vi "graphic_tester.vi"(11 "manager_daemon":refnum<class "manager_daemon.lvclass">=refnum) -> ()   [LabVIEW 2024]
uses:
  volume.type.colors--cluster.ctl
  comic_manager/manager_daemon/manager_daemon.lvclass
  selection_dropdown/Typedefs/Selection Dropdown.ctl
  selection_dropdown/selection_dropdown.lvclass/selection_dropdown.ctl
  <vilib>/Utility/miscctls.llb/LVPoint32TypeDef.ctl
  volume.object--cluster.ctl
  definitions/volume.type--enum.ctl
  comic_manager/TypeDefs/issue.display--cluster.ctl
  picture.data--cluster.ctl
  selection_dropdown/selection_dropdown.lvclass
  comic_manager/manager_daemon/manager_daemon.lvclass/manager_daemon.ctl
  comic_manager/TypeDefs/graphic.filter--cluster.ctl
  <vilib>/addons/_JKI Toolkits/State Machine/_JKI_lib_State_Machine.llb/Select State(s)_err__jki_lib_state_machine.vi
  <vilib>/addons/_JKI Toolkits/State Machine/_JKI_lib_State_Machine.llb/Periodic Trigger__ogtk__JKI-SM__jki_lib_state_machine.vi
panel:
  in  "concept filter":T1
  in  "storyArc filter":T1
  in  "character filter":T1
  in  "team filter":T1
  in  "Show Issues":bool=TRUE
  in  "Apply Filters":enum32{"AND", "OR"}(radio)
  in  "clear title":bool
  in  "title":string[](array[string])=["x-men", "x-factor", "x-force", "new mutants"]
  in  "Step Size":enum32{"Monthly", "Yearly"}(radio)
  in  "Show Legend":bool=TRUE
  in  "inc year":bool
  in  "dec year":bool
  in  "dec end year":bool
  in  "dec start year":bool
  in  "inc start year":bool
  in  "inc end year":bool
  in  "Legend":T2={"ongoing"=34559, "Limited Series"=35193, "Annuals"=16754450, "One Shots"=7566195, "Reprints"=16722176, "Star"=49407, "Epic"=8733439}
  in  "Plot End":timestamp=timestamp(3821234400 s since 1904-01-01) format="%<%x>T"
  in  "Plot Start":timestamp=timestamp(3537151200 s since 1904-01-01) format="%<%x>T"
  in  "Show All":bool=TRUE
  in  "Volume Type":T3={"Ongoing"=TRUE, "Limited Series"=TRUE, "Annuals"=TRUE, "One Shots"=TRUE, "Reference/Reprints"=TRUE, "Star Comics"=TRUE, "Epic Comics"=TRUE}
  out "volume":string
  out "found":i32=116
  in  "Exit":bool
  out "2D Picture":picture
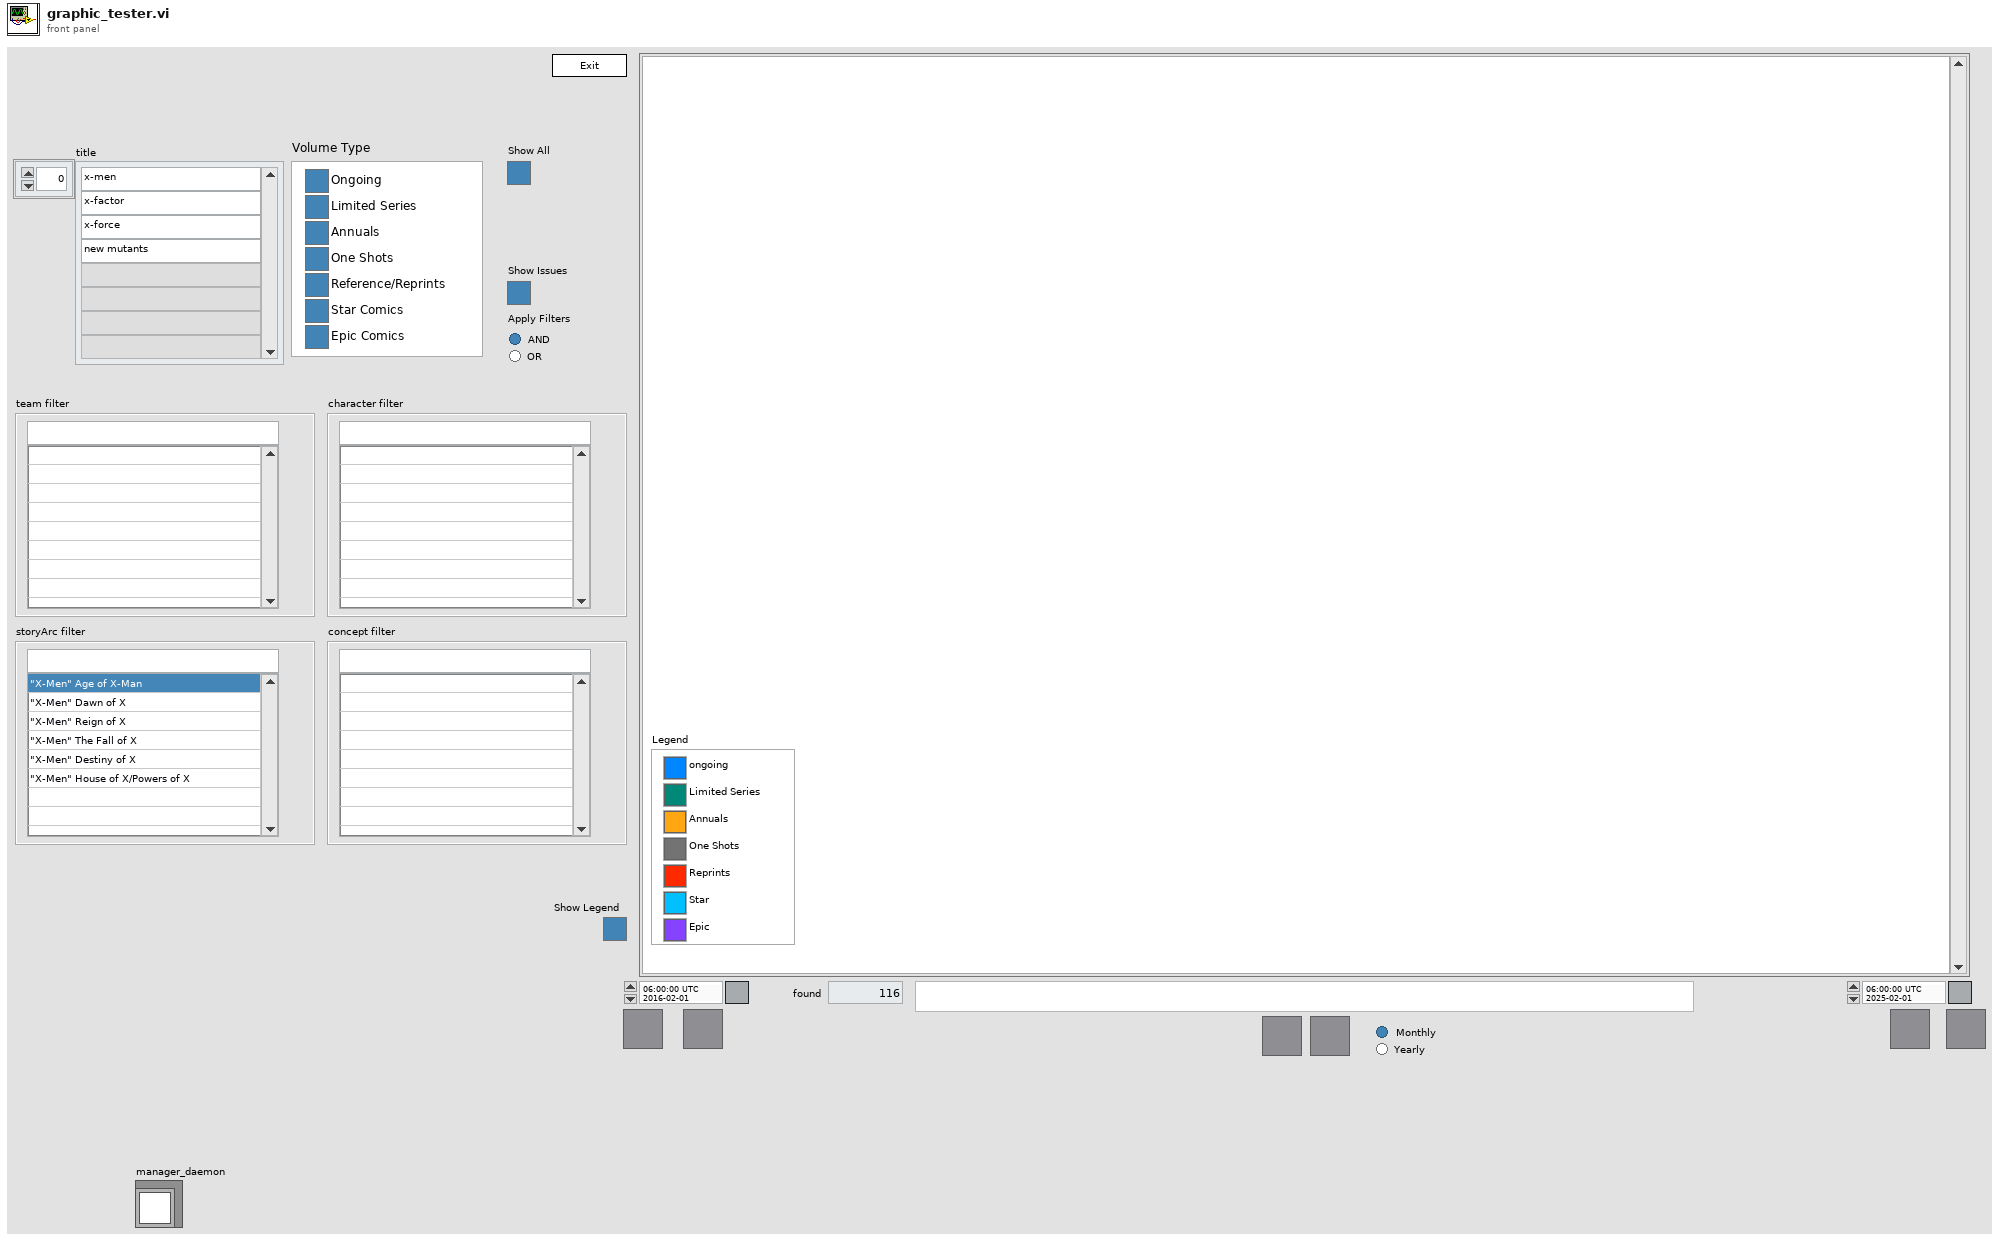
[diagram p1: front panel]
types:
  T1 = typedef "selection_dropdown.lvclass/Selection Dropdown.ctl" = cluster{"delete":bool, "available":i32, "list":i32, "cancel":bool, "selection":string, "delete all":bool}
  T2 = typedef "volume.type.colors--cluster.ctl" = cluster{"ongoing":u32, "Limited Series":u32, "Annuals":u32, "One Shots":u32, "Reprints":u32, "Star":u32, "Epic":u32}
  T3 = cluster{"Ongoing":bool, "Limited Series":bool, "Annuals":bool, "One Shots":bool, "Reference/Reprints":bool, "Star Comics":bool, "Epic Comics":bool}
  T4 = enum32{"Invalid", "Standard", "Closed", "Hidden", "Minimized", "Maximized"}
  T5 = enum32{"invalid app kind", "Development System", "Run Time System", "Student Edition", "Embedded LabVIEW", "Evaluation", "Custom"}
  T6 = typedef "graphic.filter--cluster.ctl" = cluster{"Volume Type":cluster{"Ongoing":bool, "Limited Series":bool, "Annuals":bool, "One Shots":bool, "Reference/Reprints":bool, "Star Comics":bool, "Epic Comics":bool}, "team":string[], "characters":string[], "storyArcs":string[], "Plot End":timestamp, "Plot Start":timestamp, "title":string[], "colors":T2, "concept":string[], "show all":bool, "Search by Title":enum32{"AND", "OR"}}
  T7 = cluster{"left":i16, "top":i16, "right":i16, "bottom":i16}
  T8 = typedef "volume.object--cluster.ctl" = cluster{"start date":timestamp, "end date":timestamp, "sortable_name":string, "color":u32, "volume type":T9, "issues":T10[]}
  T9 = typedef "volume.type--enum.ctl" = enum16{"Ongoing", "Limited Series", "Annual", "One Shot", "Reprint/Document", "Star Comics", "Epic Comics"}
  T10 = typedef "issue.display--cluster.ctl" = cluster{"cover_date":timestamp, "id":i32, "number":string, "fill":bool}
  T11 = typedef "picture.data--cluster.ctl" = cluster{"names":string[], "colors":u32[], "cells":cluster{"left":i16, "top":i16, "right":i16, "bottom":i16}[], "end date":timestamp, "start date":timestamp}
  T12 = typedef "LVPoint32TypeDef.ctl" = cluster{"Horizontal":i32, "Vertical":i32}
  T13 = cluster{"Core":cluster{"Current VI Reference":refnum<vi>, "Close Panel on Exit?":bool}, "volume objects":cluster{"Array":T8[]}[], "picture data":T11, "picture":picture, "rows":cluster{"left":i16, "top":i16, "right":i16, "bottom":i16}[], "cursor":T12, "manager_daemon":refnum<class "manager_daemon.lvclass">, "filters":cluster{"team filter":refnum<class "selection_dropdown.lvclass">, "story filter":refnum<class "selection_dropdown.lvclass">, "char filter":refnum<class "selection_dropdown.lvclass">, "concept filter":refnum<class "selection_dropdown.lvclass">}}
  T14 = typedef "LVPositionTypeDef.ctl" = cluster{"Left":i32, "Top":i32}
  T15 = cluster{"team filter":refnum<class "selection_dropdown.lvclass">, "story filter":refnum<class "selection_dropdown.lvclass">, "char filter":refnum<class "selection_dropdown.lvclass">, "concept filter":refnum<class "selection_dropdown.lvclass">}
  T16 = cluster{"left":i16, "top":i16, "right":i16, "bottom":i16}[]
  T17 = cluster{"Current VI Reference":refnum<vi>, "Close Panel on Exit?":bool}
  T18 = cluster{"team filter event":refnum<user-event>, "story filter event":refnum<user-event>, "char filter event":refnum<user-event>, "concept filter event":refnum<user-event>}
  T19 = typedef "LVBoundsTypeDef.ctl" = cluster{"Width":u32, "Height":u32}
  T20 = typedef "LVPointTypeDef.ctl" = cluster{"Horizontal":i16, "Vertical":i16}
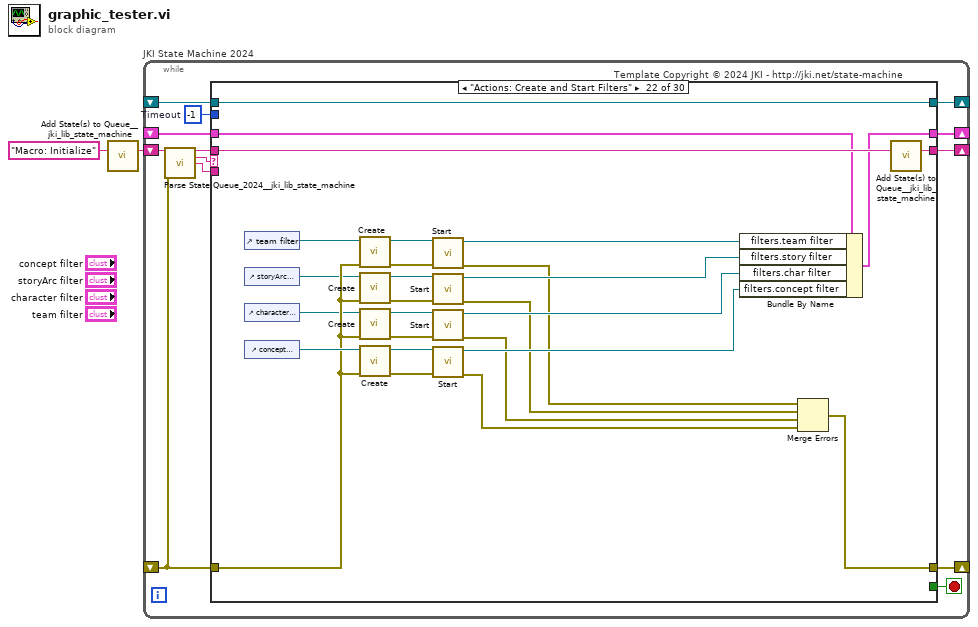
[diagram p0: block diagram]
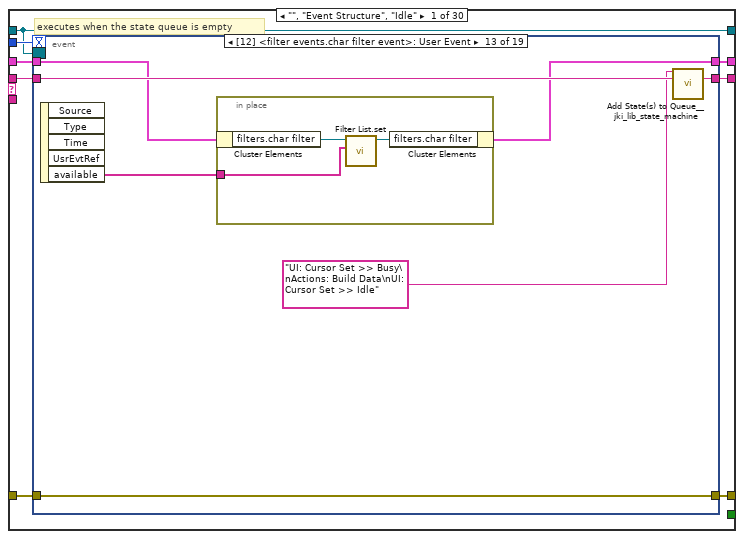
[diagram p2: hidden frame]
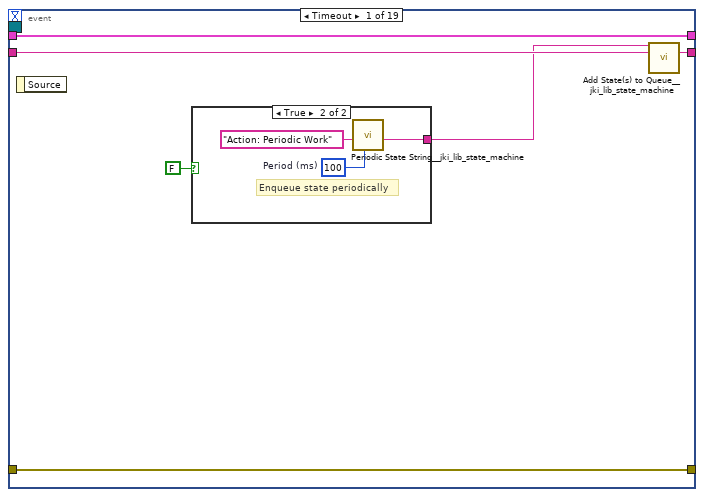
[diagram p3: hidden frame]
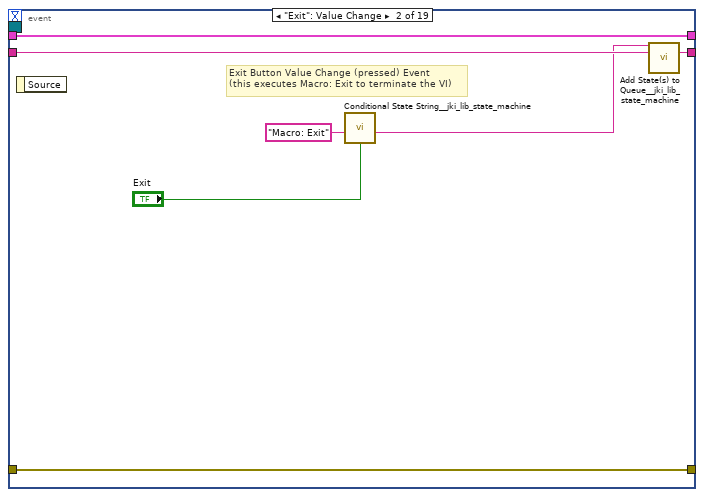
[diagram p5: hidden frame]
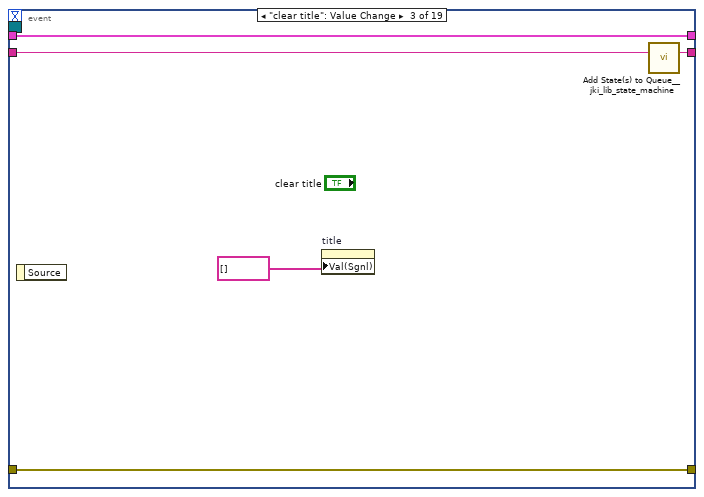
[diagram p6: hidden frame]
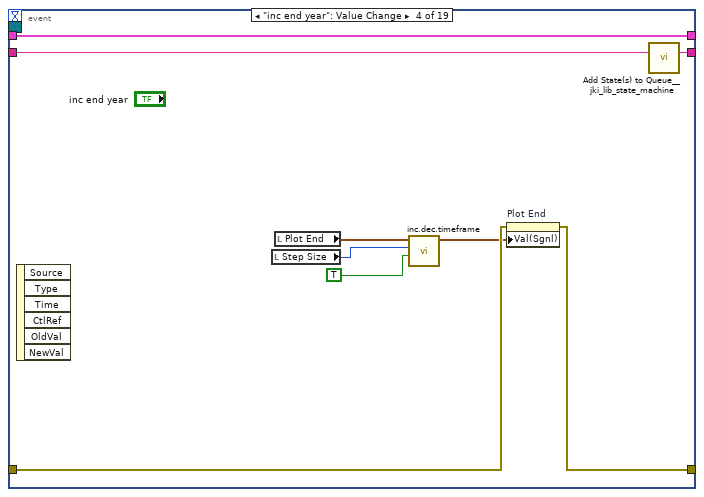
[diagram p7: hidden frame]
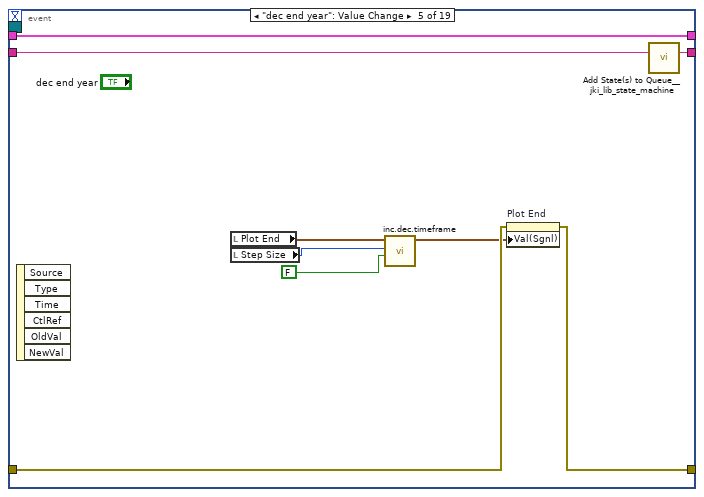
[diagram p8: hidden frame]
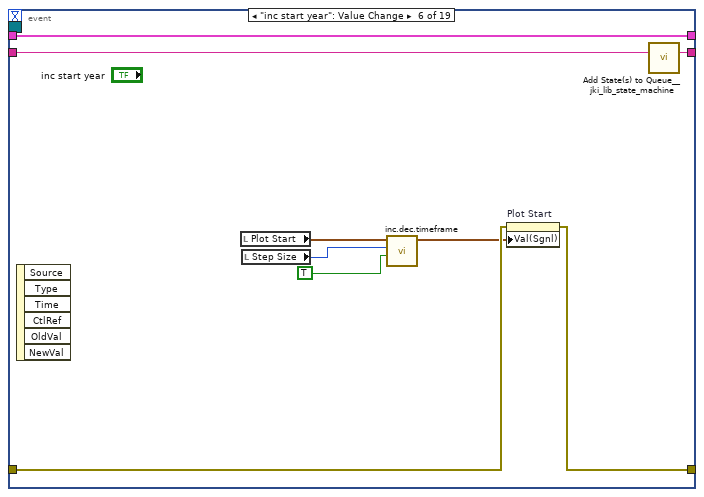
[diagram p9: hidden frame]
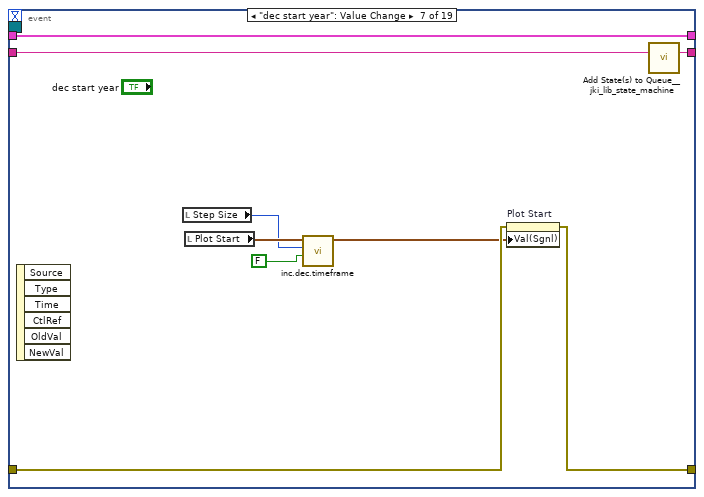
[diagram p10: hidden frame]
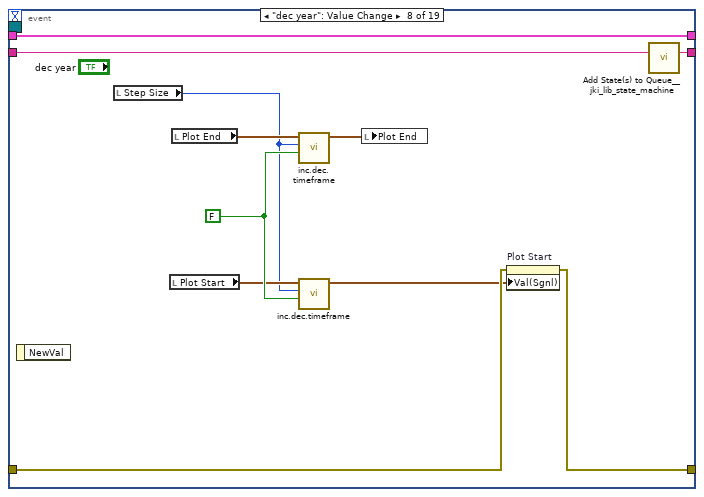
[diagram p11: hidden frame]
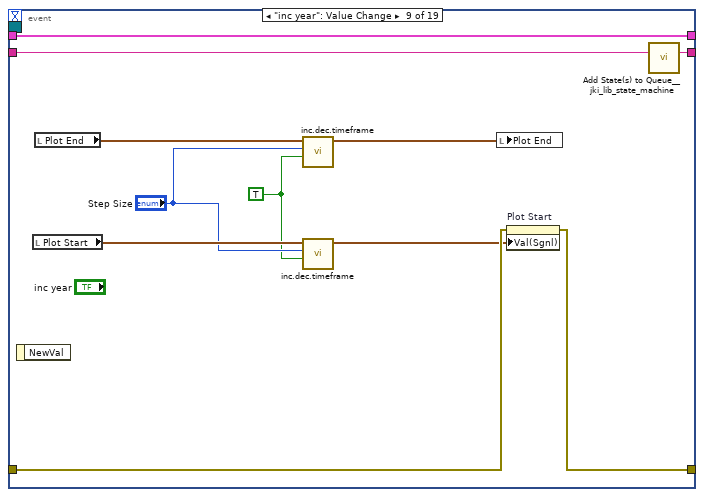
[diagram p12: hidden frame]
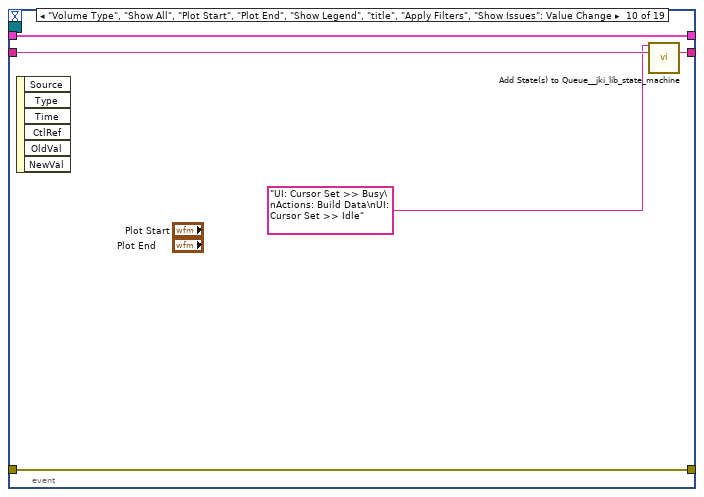
[diagram p13: hidden frame]
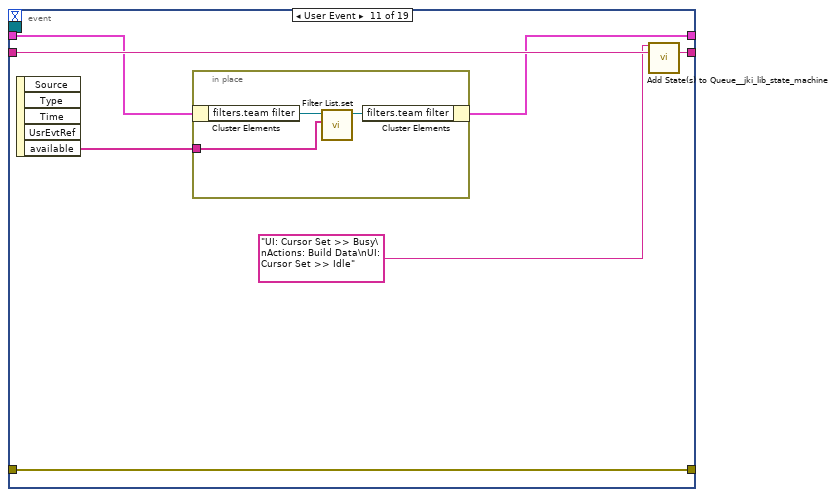
[diagram p14: hidden frame]
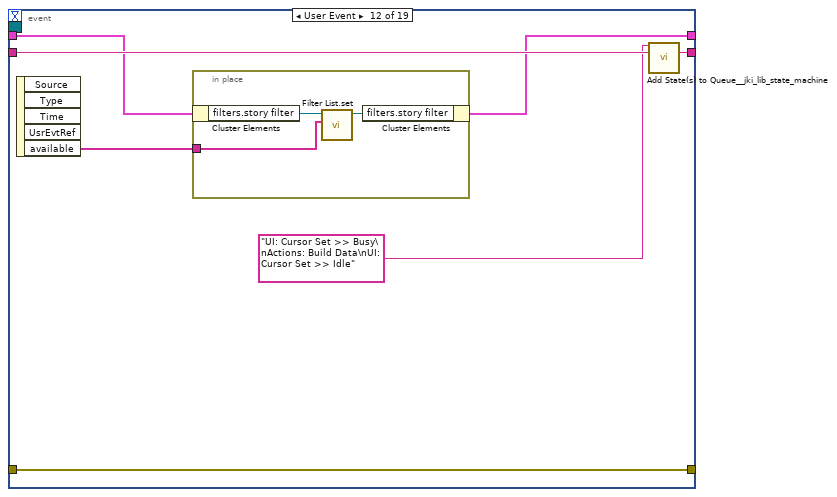
[diagram p15: hidden frame]
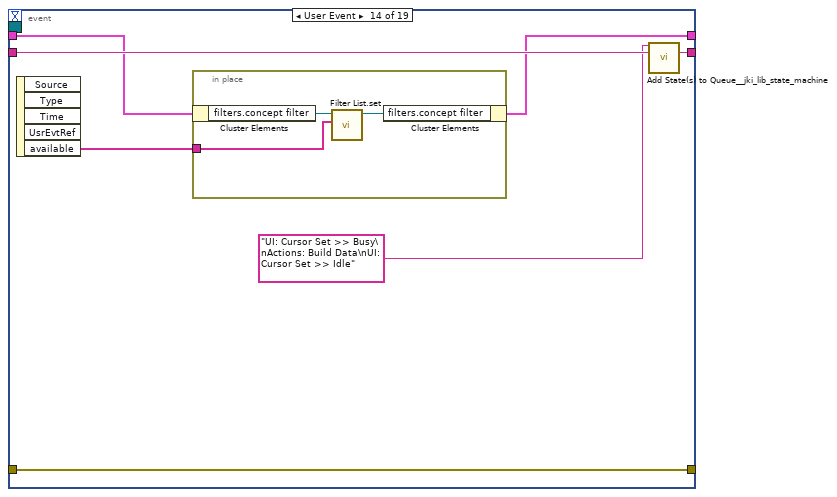
[diagram p16: hidden frame]
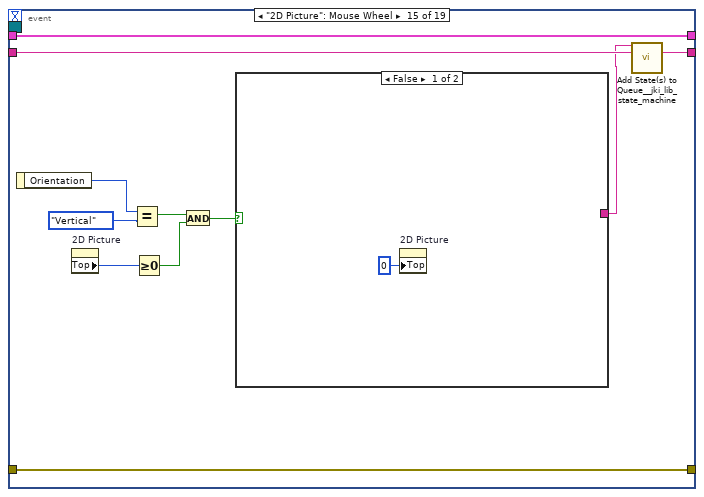
[diagram p17: hidden frame]
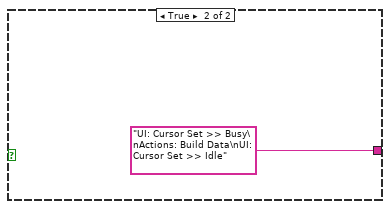
[diagram p18: hidden frame]
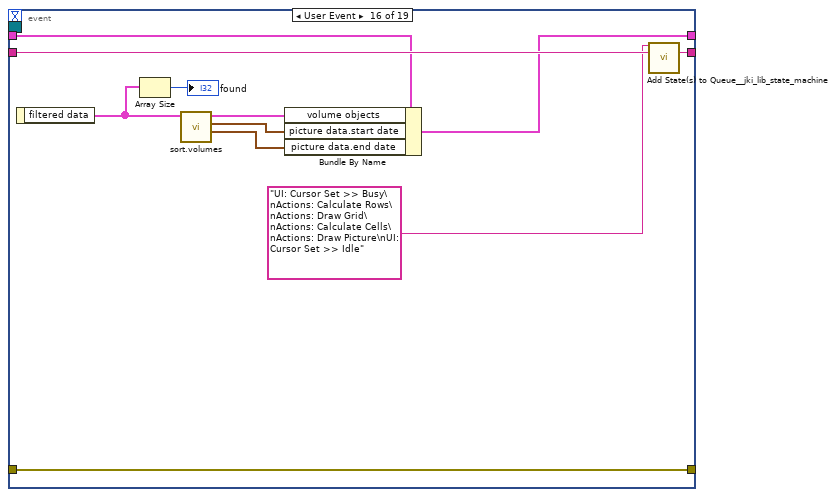
[diagram p19: hidden frame]
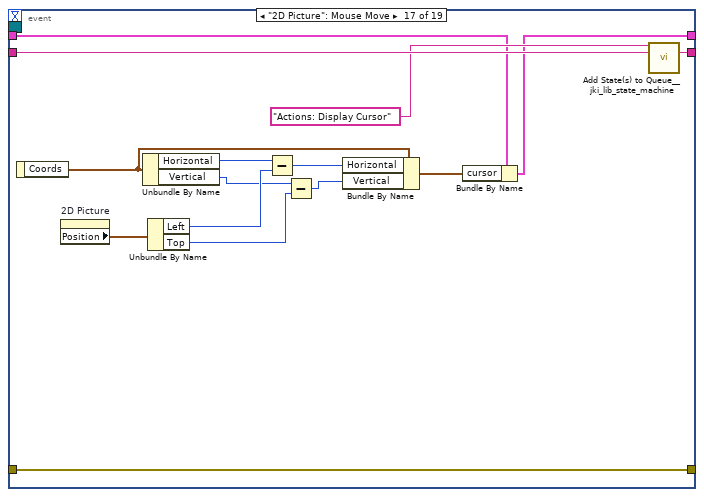
[diagram p20: hidden frame]
diagram:
  n1 = call <vilib>:"Add State(s) to Queue__jki_lib_state_machine.vi"("State(s) in (\"\")"="Macro: Initialize") -> ("States Out"=w2:string)  [unwired: 14 in]
  n2 = while "JKI State Machine 2024" {
    shift-right: [w8] -> _
    shift-left: _ -> [w7]
    shift-right: [w11] -> _
    shift-left: _ -> [w5]
    shift-right: [w10] -> _
    shift-left: w2 -> [w12]
    shift-right: [w4] -> _
    shift-left: _ -> [w3]
    stop <- w9 stop-if-true
    w6 = -1  # Timeout
    # "Template Copyright © 2024 JKI - http://jki.net/state-machine"
    n3 = call <vilib>:"Parse State Queue_2024__jki_lib_state_machine.vi"("State Queue"=w12, "Error In (no error)"=w5) -> ("Remaining States"=w14:string, "Current State"=w15:string, "Arguments"=w13:string)  [unwired: 11 in]
    n4 = case shown="\"Actions: Create and Start Filters\"" w15 {
      selector: w15 -> [_ _ w213 _ _ _ _ _ _ _ _ _ _ _ _ _ _ _ _ _ _ _ _ _ _ _ _ _ _ _]
      tunnel: w14 -> [w23 w211 w217 w237 w248 w258 w263 w281 w297 w302 w323 w329 w334 w339 w344 w351 w363 w433 w439 w449 w454 w481 w488 w497 w509 w521 w540 w565 w579 w603]
      tunnel: w13 -> [_ _ _ _ w243 _ _ _ _ _ _ _ _ _ _ w346 w357 _ _ _ _ _ _ _ _ _ _ _ _ _]
      tunnel: w7 -> [w21 w208 w215 w230 w245 w256 w260 _ w294 w299 w315 w327 w331 w337 w342 w349 w359 w430 w436 w447 w451 w465 w485 w495 w507 w518 w538 w556 w573 w594]
      tunnel: [w20 w209 w219 w234 errorcluster {"status"=FALSE, "code"=0, "source"=""} ("error out") w255 w261 w278 w287 w300 w316 w324 w332 w336 w341 w347 w360 w431 w437 w444 w452 w474 w482 w492 w504 w519 w535 w555 w577 w602] -> w11
      tunnel: w5 -> [w17 w209 w218 w234 w244 w255 w261 w278 w288 w300 w318 w325 w332 w336 w341 w348 w361 w431 w437 w444 w452 w466 w483 w494 w506 w519 w536 w554 w577 w602]
      tunnel: [w22 w210 w216 w236 w247 w257 w262 w280 w296 w301 w322 w328 w333 w338 w343 w350 w362 w432 w438 w448 w453 w480 w487 w496 w508 w520 w539 w564 w578 w603] -> w10
      tunnel: [_ _ _ _ _ TRUE _ _ _ _ _ _ _ _ _ _ _ _ _ _ _ _ _ _ _ _ _ _ _ _] -> w9
      tunnel: [w19 w208 w215 w235 w245 w256 w260 w279 w294 w299 w315 w327 w331 w337 w342 w349 w359 w430 w436 w447 w451 w475 w484 w495 w502 w518 w538 w556 w572 w593] -> w8
      tunnel: w6 -> [w18 _ _ _ _ _ _ _ _ _ _ _ _ _ _ _ _ _ _ _ _ _ _ _ _ _ _ _ _ _]
      tunnel: [w16 w207 w212 w224 w238 w253 w259 w271 w293 w298 w319 w326 w330 w335 w340 w345 w356 w429 w434 w440 w450 w479 w486 w489 w499 w510 w534 w558 w570 w589] -> w4
      tunnel: w3 -> [w16 w207 w212 w224 w238 w253 w259 w271 w293 w298 _ w326 w330 w335 w340 w345 w356 w429 w434 w440 w450 w479 w486 w489 w499 w510 w534 w558 w570 w589]
      frame "", "Event Structure", "Idle" {
        # "executes when the state queue is empty"
        n5 = event shown="[12] <filter events.char filter event>: User Event" {
          selector: w16 -> [_ _ _ _ _ _ _ _ _ _ _ _ _ _ _ _ _ _ _]
          dyn-events: _ -> [_ _ _ _ _ _ _ _ _ _ _ _ _ _ _ _ _ _ _]
          timeout: w18 -> [_ _ _ _ _ _ _ _ _ _ _ _ _ _ _ _ _ _ _]
          tunnel: w23 -> [w29 w39 w44 w53 w62 w71 w80 w91 w102 w107 w114 w124 w134 w144 w157 w171 w186 w194 w206]
          tunnel: [w28 w38 w43 w52 w61 w70 w79 w90 w101 w106 w113 w123 w133 w143 w156 w170 w185 w193 w205] -> w22
          tunnel: w21 -> [w26 w36 w41 w51 w60 w69 w78 w89 w100 w103 w109 w119 w129 w139 w158 w167 w174 w191 w203]
          tunnel: [w27 w37 w42 w49 w58 w67 w76 w87 w98 w105 w112 w122 w132 w142 w155 w169 w184 w190 w204] -> w20
          tunnel: w17 -> [w27 w37 w42 w50 w59 w68 w77 w88 w99 w105 w112 w122 w132 w142 w155 w169 w184 w189 w204]
          tunnel: [w26 w36 w41 w51 w60 w69 w78 w89 w100 w103 w110 w120 w130 w140 w158 w166 w173 w191 w203] -> w19
          event Timeout {
            n6 = event-data() -> ()  [unwired: 1 in, 1 out]
            n7 = case shown="True" FALSE {
              tunnel: [_ w32] -> w25
              frame False {
              }
              frame True {
                w30 = u32 100  # Period (ms)
                # "Enqueue state periodically"
                n8 = call <vilib>:"Periodic State String__jki_lib_state_machine.vi"("Period (ms)"=w30, "State"="Action: Periodic Work") -> ("State Out"=w32:string)  [unwired: 9 in]
              }
            }
            n9 = call <vilib>:"Add State(s) to Queue__jki_lib_state_machine.vi"("State(s) in Front (\"\")"=w25, "State(s) in (\"\")"=w29) -> ("States Out"=w28:string)  [unwired: 13 in]
          }
          event "Exit": Value Change {
            # "Exit Button Value Change (pressed) Event\n(this executes Macro: Exit to terminate the VI)"
            n10 = event-data() -> ()  [unwired: 1 in, 1 out]
            n11 = call <vilib>:"Conditional State String__jki_lib_state_machine.vi"("Do State(s)?"="Exit", "State"="Macro: Exit") -> ("State Out"=w33:string)  [unwired: 7 in]
            n12 = call <vilib>:"Add State(s) to Queue__jki_lib_state_machine.vi"("State(s) in Front (\"\")"=w33, "State(s) in (\"\")"=w39) -> ("States Out"=w38:string)  [unwired: 13 in]
          }
          event "clear title": Value Change {
            n13 = event-data() -> ()  [unwired: 1 in, 1 out]
            n14 = property on="title" class="Arr (strict)"("Val(Sgnl)"=string[] []) -> ()  [unwired: 2 in, 2 out]
            n15 = call <vilib>:"Add State(s) to Queue__jki_lib_state_machine.vi"("State(s) in (\"\")"=w44) -> ("States Out"=w43:string)  [unwired: 14 in]
          }
          event "inc end year": Value Change {
            n16 = event-data() -> ()  [unwired: 1 in, 6 out]
            n17 = local read "Step Size"() -> (w46:enum32{"Monthly", "Yearly"})
            n18 = local read "Plot End"() -> (w48:timestamp)
            n19 = call "inc.dec.timeframe.vi"("inc (T)"=TRUE, "Step Size"=w46, "Plot End"=w48) -> ("time stamp"=w47:timestamp)  [unwired: 8 in]
            n20 = property on="Plot End" class="AbsTime (strict)"(error in=w50, "Val(Sgnl)"=w47) -> (error out=w49:errorcluster)  [unwired: 1 in, 1 out]
            n21 = call <vilib>:"Add State(s) to Queue__jki_lib_state_machine.vi"("State(s) in (\"\")"=w53) -> ("States Out"=w52:string)  [unwired: 14 in]
          }
          event "dec end year": Value Change {
            n22 = event-data() -> ()  [unwired: 1 in, 6 out]
            n23 = local read "Plot End"() -> (w57:timestamp)
            n24 = local read "Step Size"() -> (w55:enum32{"Monthly", "Yearly"})
            n25 = call "inc.dec.timeframe.vi"("inc (T)"=FALSE, "Step Size"=w55, "Plot End"=w57) -> ("time stamp"=w56:timestamp)  [unwired: 8 in]
            n26 = property on="Plot End" class="AbsTime (strict)"(error in=w59, "Val(Sgnl)"=w56) -> (error out=w58:errorcluster)  [unwired: 1 in, 1 out]
            n27 = call <vilib>:"Add State(s) to Queue__jki_lib_state_machine.vi"("State(s) in (\"\")"=w62) -> ("States Out"=w61:string)  [unwired: 14 in]
          }
          event "inc start year": Value Change {
            n28 = event-data() -> ()  [unwired: 1 in, 6 out]
            n29 = local read "Plot Start"() -> (w66:timestamp)
            n30 = local read "Step Size"() -> (w64:enum32{"Monthly", "Yearly"})
            n31 = call "inc.dec.timeframe.vi"("inc (T)"=TRUE, "Step Size"=w64, "Plot End"=w66) -> ("time stamp"=w65:timestamp)  [unwired: 8 in]
            n32 = property on="Plot Start" class="AbsTime (strict)"(error in=w68, "Val(Sgnl)"=w65) -> (error out=w67:errorcluster)  [unwired: 1 in, 1 out]
            n33 = call <vilib>:"Add State(s) to Queue__jki_lib_state_machine.vi"("State(s) in (\"\")"=w71) -> ("States Out"=w70:string)  [unwired: 14 in]
          }
          event "dec start year": Value Change {
            n34 = event-data() -> ()  [unwired: 1 in, 6 out]
            n35 = local read "Step Size"() -> (w73:enum32{"Monthly", "Yearly"})
            n36 = local read "Plot Start"() -> (w75:timestamp)
            n37 = call "inc.dec.timeframe.vi"("inc (T)"=FALSE, "Step Size"=w73, "Plot End"=w75) -> ("time stamp"=w74:timestamp)  [unwired: 8 in]
            n38 = property on="Plot Start" class="AbsTime (strict)"(error in=w77, "Val(Sgnl)"=w74) -> (error out=w76:errorcluster)  [unwired: 1 in, 1 out]
            n39 = call <vilib>:"Add State(s) to Queue__jki_lib_state_machine.vi"("State(s) in (\"\")"=w80) -> ("States Out"=w79:string)  [unwired: 14 in]
          }
          event "dec year": Value Change {
            w84 = FALSE ("inc (T)")
            n40 = event-data() -> ()  [unwired: 1 in, 1 out]
            n41 = local read "Step Size"() -> (w81:enum32{"Monthly", "Yearly"})
            n42 = local read "Plot Start"() -> (w83:timestamp)
            n43 = local read "Plot End"() -> (w86:timestamp)
            n44 = call "inc.dec.timeframe.vi"("inc (T)"=w84, "Step Size"=w81, "Plot End"=w86) -> ("time stamp"=w85:timestamp)  [unwired: 8 in]
            n45 = call "inc.dec.timeframe.vi"("inc (T)"=w84, "Step Size"=w81, "Plot End"=w83) -> ("time stamp"=w82:timestamp)  [unwired: 8 in]
            n46 = local write "Plot End"(w85) -> ()
            n47 = property on="Plot Start" class="AbsTime (strict)"(error in=w88, "Val(Sgnl)"=w82) -> (error out=w87:errorcluster)  [unwired: 1 in, 1 out]
            n48 = call <vilib>:"Add State(s) to Queue__jki_lib_state_machine.vi"("State(s) in (\"\")"=w91) -> ("States Out"=w90:string)  [unwired: 14 in]
          }
          event "inc year": Value Change {
            w92 = TRUE ("inc (T)")
            n49 = event-data() -> ()  [unwired: 1 in, 1 out]
            n50 = local read "Plot Start"() -> (w95:timestamp)
            n51 = local read "Plot End"() -> (w97:timestamp)
            n52 = call "inc.dec.timeframe.vi"("inc (T)"=w92, "Step Size"="Step Size", "Plot End"=w97) -> ("time stamp"=w96:timestamp)  [unwired: 8 in]
            n53 = call "inc.dec.timeframe.vi"("inc (T)"=w92, "Step Size"="Step Size", "Plot End"=w95) -> ("time stamp"=w94:timestamp)  [unwired: 8 in]
            n54 = local write "Plot End"(w96) -> ()
            n55 = property on="Plot Start" class="AbsTime (strict)"(error in=w99, "Val(Sgnl)"=w94) -> (error out=w98:errorcluster)  [unwired: 1 in, 1 out]
            n56 = call <vilib>:"Add State(s) to Queue__jki_lib_state_machine.vi"("State(s) in (\"\")"=w102) -> ("States Out"=w101:string)  [unwired: 14 in]
          }
          event "Volume Type", "Show All", "Plot Start", "Plot End", "Show Legend", "title", "Apply Filters", "Show Issues": Value Change {
            n57 = event-data() -> ()  [unwired: 1 in, 6 out]
            n58 = call <vilib>:"Add State(s) to Queue__jki_lib_state_machine.vi"("State(s) in Front (\"\")"="UI: Cursor Set >> Busy\nActions: Build Data\nUI: Cursor Set >> Idle", "State(s) in (\"\")"=w107) -> ("States Out"=w106:string)  [unwired: 13 in]
          }
          event User Event {
            n59 = event-data() -> ("available"=w108:string[])  [unwired: 1 in, 4 out]
            n60 = in-place {
              in-place-border: w108 -> [w115]
              n61 = in-place-cluster #1(w109) -> ("filters.team filter"=w117:refnum<class "selection_dropdown.lvclass">)
              n62 = call "Filter List.set.vi"("filter list"=w115, "selection_dropdown in"=w117) -> ("selection_dropdown out"=w116:refnum<class "selection_dropdown.lvclass">)  [unwired: 9 in]
              n63 = in-place-cluster #1("filters.team filter"=w116) -> (w110:T13)
            }
            n64 = call <vilib>:"Add State(s) to Queue__jki_lib_state_machine.vi"("State(s) in Front (\"\")"="UI: Cursor Set >> Busy\nActions: Build Data\nUI: Cursor Set >> Idle", "State(s) in (\"\")"=w114) -> ("States Out"=w113:string)  [unwired: 13 in]
          }
          event User Event {
            n65 = event-data() -> ("available"=w118:string[])  [unwired: 1 in, 4 out]
            n66 = in-place {
              in-place-border: w118 -> [w125]
              n67 = in-place-cluster #2(w119) -> ("filters.story filter"=w127:refnum<class "selection_dropdown.lvclass">)
              n68 = call "Filter List.set.vi"("filter list"=w125, "selection_dropdown in"=w127) -> ("selection_dropdown out"=w126:refnum<class "selection_dropdown.lvclass">)  [unwired: 9 in]
              n69 = in-place-cluster #2("filters.story filter"=w126) -> (w120:T13)
            }
            n70 = call <vilib>:"Add State(s) to Queue__jki_lib_state_machine.vi"("State(s) in Front (\"\")"="UI: Cursor Set >> Busy\nActions: Build Data\nUI: Cursor Set >> Idle", "State(s) in (\"\")"=w124) -> ("States Out"=w123:string)  [unwired: 13 in]
          }
          event User Event {
            n71 = event-data() -> ("available"=w128:string[])  [unwired: 1 in, 4 out]
            n72 = in-place {
              in-place-border: w128 -> [w135]
              n73 = in-place-cluster #3(w129) -> ("filters.char filter"=w137:refnum<class "selection_dropdown.lvclass">)
              n74 = call "Filter List.set.vi"("filter list"=w135, "selection_dropdown in"=w137) -> ("selection_dropdown out"=w136:refnum<class "selection_dropdown.lvclass">)  [unwired: 9 in]
              n75 = in-place-cluster #3("filters.char filter"=w136) -> (w130:T13)
            }
            n76 = call <vilib>:"Add State(s) to Queue__jki_lib_state_machine.vi"("State(s) in Front (\"\")"="UI: Cursor Set >> Busy\nActions: Build Data\nUI: Cursor Set >> Idle", "State(s) in (\"\")"=w134) -> ("States Out"=w133:string)  [unwired: 13 in]
          }
          event User Event {
            n77 = event-data() -> ("available"=w138:string[])  [unwired: 1 in, 4 out]
            n78 = in-place {
              in-place-border: w138 -> [w145]
              n79 = in-place-cluster #4(w139) -> ("filters.concept filter"=w147:refnum<class "selection_dropdown.lvclass">)
              n80 = call "Filter List.set.vi"("filter list"=w145, "selection_dropdown in"=w147) -> ("selection_dropdown out"=w146:refnum<class "selection_dropdown.lvclass">)  [unwired: 9 in]
              n81 = in-place-cluster #4("filters.concept filter"=w146) -> (w140:T13)
            }
            n82 = call <vilib>:"Add State(s) to Queue__jki_lib_state_machine.vi"("State(s) in Front (\"\")"="UI: Cursor Set >> Busy\nActions: Build Data\nUI: Cursor Set >> Idle", "State(s) in (\"\")"=w144) -> ("States Out"=w143:string)  [unwired: 13 in]
          }
          event "2D Picture": Mouse Wheel {
            n83 = event-data() -> ("Orientation"=w154:enum16{"Horizontal", "Vertical"})  [unwired: 1 in]
            n84 = property on="2D Picture" class="Pict"() -> ("Top"=w152:i16)  [unwired: 2 in, 2 out]
            n85 = Equal?(x=w154, y=enum16{"Horizontal", "Vertical"}."Vertical") -> (x = y?=w151:bool)
            n86 = Greater Or Equal To 0?(x=w152) -> (x >= 0?=w150:bool)
            n87 = And(x=w151, y=w150) -> (x .and. y?=w149:bool)
            n88 = case shown="False" w149 {
              tunnel: [_ "UI: Cursor Set >> Busy\nActions: Build Data\nUI: Cursor Set >> Idle"] -> w148
              frame False {
                n89 = property on="2D Picture" class="Pict"("Top"=i16 0 ("Origin:Top")) -> ()  [unwired: 2 in, 2 out]
              }
              frame True {
              }
            }
            n90 = call <vilib>:"Add State(s) to Queue__jki_lib_state_machine.vi"("State(s) in Front (\"\")"=w148, "State(s) in (\"\")"=w157) -> ("States Out"=w156:string)  [unwired: 13 in]
          }
          event User Event {
            n91 = event-data() -> ("filtered data"=w161:T8[])  [unwired: 1 in]
            n92 = Array Size(array=w161) -> (size(s)=→"found":i32)
            n93 = call "sort.volumes.vi"("volumes"=w161) -> ("end date"=w163:timestamp, "start date"=w164:timestamp, "volumes by row"=w165:cluster{"Array":T8[]}[])  [unwired: 8 in]
            n94 = Bundle By Name(cluster=w167, "volume objects"=w165, "picture data.start date"=w164, "picture data.end date"=w163) -> (w166:T13)
            n95 = call <vilib>:"Add State(s) to Queue__jki_lib_state_machine.vi"("State(s) in Front (\"\")"="UI: Cursor Set >> Busy\nActions: Calculate Rows\nActions: Draw Grid\nActions: Calculate Cells\nActions: Draw Picture\nUI: Cursor Set >> Idle", "State(s) in (\"\")"=w171) -> ("States Out"=w170:string)  [unwired: 13 in]
          }
          event "2D Picture": Mouse Move {
            n96 = event-data() -> ("Coords"=w178:T12)  [unwired: 1 in]
            n97 = property on="2D Picture" class="Pict"() -> ("Position"=w183:T14)  [unwired: 2 in, 2 out]
            n98 = Unbundle By Name(w178) -> ("Horizontal"=w182:i32, "Vertical"=w180:i32)
            n99 = Unbundle By Name(w183) -> ("Left"=w181:i32, "Top"=w179:i32)
            n100 = Subtract(x=w182, y=w181) -> (x-y=w177:i32)
            n101 = Subtract(x=w180, y=w179) -> (x-y=w176:i32)
            n102 = Bundle By Name(cluster=w178, "Horizontal"=w177, "Vertical"=w176) -> (w172:T12)
            n103 = Bundle By Name(cluster=w174, "cursor"=w172) -> (w173:T13)
            n104 = call <vilib>:"Add State(s) to Queue__jki_lib_state_machine.vi"("State(s) in Front (\"\")"="Actions: Display Cursor" ("State(s) in Front (\"\")"), "State(s) in (\"\")"=w186) -> ("States Out"=w185:string)  [unwired: 13 in]
          }
          event "2D Picture": Mouse Down? {
            n105 = event-data() -> ("Coords"=w192:T12, "Mods.Double Click"=w187:bool)  [unwired: 1 in]
            n106 = case shown="True" w187 {
              tunnel: w192 -> [_ _]
              tunnel: w191 -> [_ w200]
              tunnel: w189 -> [w195 w197]
              tunnel: [w195 w196] -> w190
              frame False {
              }
              frame True {
                n107 = Unbundle By Name(w200) -> ("manager_daemon"=w199:refnum<class "manager_daemon.lvclass">)
                n108 = local read "volume"() -> (w198:string)
                n109 = call "display info.vi"("error in (no error)"=w197, "volume name"=w198, "manager_daemon in"=w199) -> ("error out"=w196:errorcluster)  [unwired: 7 in, 1 out]
              }
            }
            n110 = event-data("Discard?"=TRUE) -> ()  [unwired: 4 in, 1 out]
            n111 = call <vilib>:"Add State(s) to Queue__jki_lib_state_machine.vi"("State(s) in (\"\")"=w194) -> ("States Out"=w193:string)  [unwired: 14 in]
          }
          event Panel Close? {
            # "Discard the event because we'll close the front panel ourselves in Macro: Exit"
            # "Close Panel button (pressed) Event\n(this executes Macro: Exit to terminate the VI)"
            n112 = event-data() -> ()  [unwired: 1 in, 1 out]
            n113 = event-data("Discard?"=TRUE) -> ()  [unwired: 1 in, 1 out]
            n114 = call <vilib>:"Add State(s) to Queue__jki_lib_state_machine.vi"("State(s) in Front (\"\")"="Macro: Exit", "State(s) in (\"\")"=w206) -> ("States Out"=w205:string)  [unwired: 13 in]
          }
        }
      }
      frame "---------- Core ----------" {
        # "Do not put any code in this frame.\n(it is a separator no-op)"
        n115 = call <vilib>:"Add State(s) to Queue__jki_lib_state_machine.vi"("State(s) in (\"\")"=w211) -> ("States Out"=w210:string)  [unwired: 14 in]
      }
      frame Default {
        w222 = 42 items=["No error", "Argument error", "Memory is full", "Out of zone", "End of file", "File already open", "Generic file I/O error", "File not found", "File permission error", "Disk is full", "Duplicate path", "Too many files open", "System feature not enabled", "Resource file not found", "Cannot add resource", "Resource not found", "Image not found", "Image memory error", "Pen does not exist", "Config type invalid", "Config token not found", "Config parse error", "Config memory error", "Bad external code format", "Bad external code offset", "External code not present", "Null window", "Destroy window error", "Null menu", "Print aborted", "Bad print record", "Print driver error", "Windows error during printing", "Memory error during printing", "Print dialog error", "Generic print error", "Invalid device refnum", "Device not found", "Device parameter error", "Device unit error", "Cannot open device", "Device call aborted", "Generic error", "Cancelled by user", "Object ID too low", "Object ID too high", "Object not in heap", "Unknown heap", "Unknown object (invalid DefProc)", "Unknown object (DefProc not in table)", "Message out of range", "Invalid (null) method", "Unknown message", "Manager call not supported", "Bad address", "Network operation in progress", "Network operation timed out", "Connection is busy", "Network attribute not supported", "Network error", "Address in use", "System out of memory", "Connection aborted", "Connection refused", "Not connected", "Already connected", "Connection closed", "Initialization error (interapplication manager)", "Bad occurrence", "Wait on unbound occurrence handler", "Occurrence queue overflow", "Datalog type conflict", "Unused", "Unrecognized type (interapplication manager)", "Memory corrupt", "Failed to make temporary DLL", "Old CIN version", "Drag socket not found", "Failed to load drop-object", "Failed to register OLE object", "Failed to release OLE object", "Format specifier type mismatch", "Unknown format specifier", "Too few format specifiers", "Too many format specifiers", "Scan failed", "Newer CIN version", "Error converting to variant", "Runtime menu error", "Password tampered", "Variant attribute not found", "Incompatible variant data type", "Event data is not available", "Event Store is not present", "Occurrence is not found", "Event Queue is not created", "Event info is not available", "Refnum passed is NULL", "Error retrieving Class GUID", "Error retrieving CoClass GUID", "Error retrieving TypeLib GUID.", "Bad built application magic bytes.", "Specific driver is different from the specific driver associated with the Logical Name.", "There is no session opened to the class driver.", "Max Error", "MAX - Error with config objects", "MAX - Error loading configuration", "MAX - Group not supported"]
        # "Current State"
        # "Do not delete, rename, or modify this frame.\n(this is used to capture unhandled states and typos)"
        # "Handle mistyped state name (developer tool)"
        n116 = Format Into String(format string="Software Exception: Unhandled State \"%s\"." ("message"), error in=w218, w213) -> (resulting string=w221:string, error out=w220:errorcluster)  [unwired: 1 in]
        n117 = call <vilib>:"Error Cluster From Error Code.vi"("show call chain? (False)"=TRUE, "error in (no error)"=w220, "error message (\"\")"=w221, "error code (0)"=w222) -> ("error out"=w219:errorcluster)  [unwired: 5 in]
        n118 = call <vilib>:"Add State(s) to Queue__jki_lib_state_machine.vi"("State(s) in (\"\")"=w217) -> ("States Out"=w216:string)  [unwired: 14 in]
      }
      frame "Initialize Core Data" {
        # "Do not delete, rename, or modify this frame.\n(this is used to determine panel behavior on exit)"
        # "originally closed?"
        # "exe?"
        # "If panel starts closed or is an EXE, then close it when we exit"
        n119 = property class="VI"() -> ("FP.State"=w227:T4)  [unwired: 2 in, 2 out]
        n120 = property class="App"() -> ("App.Kind"=w233:T5)  [unwired: 2 in, 2 out]
        n121 = control-ref of="Current VI Reference"() -> (w228:refnum<vi>)
        n122 = Equal?(x=w227, y=T4."Closed" ("Front Panel Window:State")) -> (x = y?=w225:bool)
        n123 = Equal?(x=w233, y=T5."Run Time System" ("Application:Kind")) -> (x = y?=w231:bool)
        n124 = Or(x=w225, y=w231) -> (x .or. y?=w229:bool)
        n125 = Bundle By Name(cluster=w230, "Core.Current VI Reference"=w228, "Core.Close Panel on Exit?"=w229) -> (w235:T13)
        n126 = call <vilib>:"Add State(s) to Queue__jki_lib_state_machine.vi"("State(s) in (\"\")"=w237) -> ("States Out"=w236:string)  [unwired: 14 in]
      }
      frame "Error Handler" {
        # "When running as sourcecode, this function will add previous state data to the error message to aid the developer in troubleshoot errors.\nIf run as an executable, no additional information is added to the error message."
        # "This state receives both Errors and Warnings which is how the Status of this wire can be FALSE"
        # "Unhandled Error -- Display it"
        # "Handle any errors or warnings here.\nYou can also output any states to clean-up after errors or warnings occur"
        # "Clear error or warning"
        n127 = disable-structure shown="Default" {
          disable-tunnel: w244 -> [w251 w252]
          disable-tunnel: w243 -> [w250 _]
          disable-tunnel: [w249 w252] -> w242
          frame condition #0 (active) {
            n128 = call <vilib>:"Append Error Details__jki_lib_state_machine.vi"("error in (no error)"=w251, "Previous State and Argument(s)"=w250) -> ("error out"=w249:errorcluster)  [unwired: 9 in]
          }
          frame condition #1 {
          }
        }
        n129 = call <vilib>:"General Error Handler.vi"("error in (no error)"=w242) -> ()  [unwired: 10 in, 5 out]
        n130 = call-poly <vilib>:"Select State(s)__jki_lib_state_machine.vi"("State(s) if True (\"\")"="/* Post Error States", "Select"=w242, "State(s) if False (\"\")"="/* Post Warning States") -> ("States Out"=w240:string)  [unwired: 12 in]
        n131 = call <vilib>:"Add State(s) to Queue__jki_lib_state_machine.vi"("State(s) in Front (\"\")"=w240, "State(s) in (\"\")"=w248) -> ("States Out"=w247:string)  [unwired: 13 in]
      }
      frame "Exit" {
        # "Do not put any code in this frame.\n(No errors that occur here will be handled.)"
        n132 = call <vilib>:"Add State(s) to Queue__jki_lib_state_machine.vi"("State(s) in (\"\")"=w258) -> ("States Out"=w257:string)  [unwired: 14 in]
      }
      frame "---------- Data ----------" {
        # "Do not put any code in this frame.\n(It is a separator no-op. You can make a copy of this frame to create a new Data frame)"
        n133 = call <vilib>:"Add State(s) to Queue__jki_lib_state_machine.vi"("State(s) in (\"\")"=w263) -> ("States Out"=w262:string)  [unwired: 14 in]
      }
      frame "Data: Initialize" {
        w265 = T15 {"team filter"=refnum, "story filter"=refnum, "char filter"=refnum, "concept filter"=refnum}  # filters
        w266 = refnum<class "selection_dropdown.lvclass"> refnum  # concept filter
        w268 = refnum<class "selection_dropdown.lvclass"> refnum  # story filter
        w267 = refnum<class "selection_dropdown.lvclass"> refnum  # char filter
        w269 = refnum<class "selection_dropdown.lvclass"> refnum  # team filter
        w272 = T11 {"names"=[], "colors"=[], "cells"=[], "end date"=timestamp(0 s since 1904-01-01), "start date"=timestamp(0 s since 1904-01-01)}  # picture data
        w273 = cluster{"Array":T8[]}[] []  # volume objects
        w274 = T12 {"Horizontal"=0, "Vertical"=0}  # cursor
        w275 = T16 []  # rows
        w276 = picture data[5B]  # picture
        w277 = T17 {"Current VI Reference"=refnum, "Close Panel on Exit?"=FALSE}  # Core
        # "Data names and types of shift register data are defined by this bundle."
        # "Initialize the shift-register data, here.\n(data names are defined by what you wire into the bundle function)"
        n134 = Bundle(cluster=w265, "team filter"=w269, "story filter"=w268, "char filter"=w267, "concept filter"=w266) -> (w264:T15)
        n135 = Bundle("Core"=w277, "volume objects"=w273, "picture data"=w272, "picture"=w276, "rows"=w275, "cursor"=w274, "manager_daemon"="manager_daemon", "filters"=w264) -> (w279:T13)  [unwired: 1 in]
        n136 = call <vilib>:"Add State(s) to Queue__jki_lib_state_machine.vi"("State(s) in (\"\")"=w281) -> ("States Out"=w280:string)  [unwired: 14 in]
      }
      frame "Data: Cleanup" {
        # "Cleanup any data and references, here.\n(this is called automatically, by the Macro: Exit)"
        n137 = Unbundle By Name(w294) -> ("Core.Current VI Reference"=w295:refnum<vi>, "filters.team filter"=w289:refnum<class "selection_dropdown.lvclass">, "filters.story filter"=w290:refnum<class "selection_dropdown.lvclass">, "filters.char filter"=w291:refnum<class "selection_dropdown.lvclass">, "filters.concept filter"=w292:refnum<class "selection_dropdown.lvclass">)
        n138 = call "Destroy.vi"("selection_dropdown in"=w292) -> ("error out"=w282:errorcluster)  [unwired: 9 in, 1 out]
        n139 = call "Destroy.vi"("selection_dropdown in"=w291) -> ("error out"=w283:errorcluster)  [unwired: 9 in, 1 out]
        n140 = call "Destroy.vi"("selection_dropdown in"=w290) -> ("error out"=w284:errorcluster)  [unwired: 9 in, 1 out]
        n141 = call "Destroy.vi"("selection_dropdown in"=w289) -> ("error out"=w285:errorcluster)  [unwired: 9 in, 1 out]
        n142 = Close Reference(reference=w295) -> (error out=w286:errorcluster)  [unwired: 1 in]
        n143 = Merge Errors(w288, w286, w285, w284, w283, w282) -> (w287:errorcluster)
        n144 = call <vilib>:"Add State(s) to Queue__jki_lib_state_machine.vi"("State(s) in (\"\")"=w297) -> ("States Out"=w296:string)  [unwired: 14 in]
      }
      frame "---------- Events ----------" {
        # "Do not put any code in this frame.\n(It is a separator no-op. You can make a copy of this frame to create a new UI frame)"
        n145 = call <vilib>:"Add State(s) to Queue__jki_lib_state_machine.vi"("State(s) in (\"\")"=w302) -> ("States Out"=w301:string)  [unwired: 14 in]
      }
      frame "Events: Register" {
        w308 = T18 {"team filter event"=refnum, "story filter event"=refnum, "char filter event"=refnum, "concept filter event"=refnum}  # filter events
        w320 = cluster{"My Event Data":bool} {"My Event Data"=FALSE}  # My User Event
        # "Do not put any code in this frame.\n(It is a separator no-op. You can make a copy of this frame to create a new UI frame)"
        n146 = Unbundle By Name(w315) -> ("manager_daemon"=w314:refnum<class "manager_daemon.lvclass">, "filters.team filter"=w312:refnum<class "selection_dropdown.lvclass">, "filters.story filter"=w311:refnum<class "selection_dropdown.lvclass">, "filters.char filter"=w310:refnum<class "selection_dropdown.lvclass">, "filters.concept filter"=w309:refnum<class "selection_dropdown.lvclass">)
        n147 = Create User Event(user event datatype=w320, error in=w318) -> (user event=w321:refnum<user-event>, error out=w317:errorcluster)
        n148 = call "filtered.data.event.get.vi"("manager_daemon in"=w314) -> ("filtered data event"=w313:refnum<user-event>)  [unwired: 9 in, 1 out]
        n149 = call "Filter List Event.get.vi"("selection_dropdown in"=w312) -> ("filter list event"=w307:refnum<user-event>)  [unwired: 9 in, 1 out]
        n150 = call "Filter List Event.get.vi"("selection_dropdown in"=w311) -> ("filter list event"=w306:refnum<user-event>)  [unwired: 9 in, 1 out]
        n151 = call "Filter List Event.get.vi"("selection_dropdown in"=w310) -> ("filter list event"=w305:refnum<user-event>)  [unwired: 9 in, 1 out]
        n152 = call "Filter List Event.get.vi"("selection_dropdown in"=w309) -> ("filter list event"=w304:refnum<user-event>)  [unwired: 9 in, 1 out]
        n153 = Bundle(cluster=w308, "team filter event"=w307, "story filter event"=w306, "char filter event"=w305, "concept filter event"=w304) -> (w303:T18)
        n154 = register-events(error in=w317, w321, w313, w303) -> (reference out=w319:refnum<event-registration>, error out=w316:errorcluster)  [unwired: 1 in]
        n155 = call <vilib>:"Add State(s) to Queue__jki_lib_state_machine.vi"("State(s) in (\"\")"=w323) -> ("States Out"=w322:string)  [unwired: 14 in]
      }
      frame "Events: Unregister" {
        # "Do not put any code in this frame.\n(It is a separator no-op. You can make a copy of this frame to create a new UI frame)"
        n156 = Unregister For Events(event registration refnum=w326, error in=w325) -> (error out=w324:errorcluster)
        n157 = call <vilib>:"Add State(s) to Queue__jki_lib_state_machine.vi"("State(s) in (\"\")"=w329) -> ("States Out"=w328:string)  [unwired: 14 in]
      }
      frame "---------- UI ----------" {
        # "Do not put any code in this frame.\n(It is a separator no-op. You can make a copy of this frame to create a new UI frame)"
        n158 = call <vilib>:"Add State(s) to Queue__jki_lib_state_machine.vi"("State(s) in (\"\")"=w334) -> ("States Out"=w333:string)  [unwired: 14 in]
      }
      frame "UI: Initialize" {
        # "Initialize the User Interface, here.\n(this is called automatically, by the Macro: Initialize)"
        n159 = call <vilib>:"Add State(s) to Queue__jki_lib_state_machine.vi"("State(s) in (\"\")"=w339) -> ("States Out"=w338:string)  [unwired: 14 in]
      }
      frame "UI: Uninitialize" {
        # "Cleanup the User Interface, here.\n(this is called automatically, by the Macro: Exit)"
        n160 = call <vilib>:"Add State(s) to Queue__jki_lib_state_machine.vi"("State(s) in (\"\")"=w344) -> ("States Out"=w343:string)  [unwired: 14 in]
      }
      frame "UI: Cursor Set" {
        # "Argument"
        # "Set and Unset Cursor Busy.\n(Usage: \"UI: Cursor Set >> Busy|Idle\")"
        n161 = case shown="\"Idle\", Default" w346 {
          tunnel: w348 -> [w353 w355]
          tunnel: [w352 w354] -> w347
          frame "Idle", Default {
            n162 = call <vilib>:"Unset Busy.vi"("error in (no error)"=w353) -> ("error out"=w352:errorcluster)  [unwired: 10 in]
          }
          frame "Busy" {
            n163 = call <vilib>:"Set Busy.vi"("error in (no error)"=w355) -> ("error out"=w354:errorcluster)  [unwired: 9 in, 1 out]
          }
        }
        n164 = call <vilib>:"Add State(s) to Queue__jki_lib_state_machine.vi"("State(s) in (\"\")"=w351) -> ("States Out"=w350:string)  [unwired: 14 in]
      }
      frame "UI: Front Panel State" {
        # "Argument"
        # "Set Front Panel Open or Closed\n(Usage: \"UI: Front Panel State >> Open|Close\")"
        n165 = Unbundle By Name(w359) -> ("Core.Current VI Reference"=w358:refnum<vi>)
        n166 = case shown="\"Minimize\", \"Minimized\"" w357 {
          tunnel: w361 -> [w369 w384 w395 w408 w421]
          tunnel: [w371 w385 w397 w410 w423] -> w360
          tunnel: w358 -> [w370 w382 w396 w409 w422]
          frame "Open", "Standard", Default {
            w364 = T4."Standard" ("State")
            n167 = property class="VI"(reference=w370, error in=w369) -> (reference out=w367:refnum<vi>, error out=w368:errorcluster, "FP.State"=w366:T4)
            n168 = Not Equal?(x=w366, y=w364) -> (x != y?=w365:bool)
            n169 = case shown="True" w365 {
              tunnel: [w375 w377] -> w371
              tunnel: w368 -> [w374 w377]
              tunnel: w367 -> [w373 _]
              tunnel: w364 -> [w372 _]
              frame True {
                n170 = invoke class="VI" method="FP.Open"(reference=w373, error in=w374, "Activate"=TRUE, "State"=w372) -> (error out=w375:errorcluster)  [unwired: 1 in, 4 out]
              }
              frame False {
              }
            }
          }
          frame "Close", "Closed" {
            n171 = property class="VI"(reference=w382, error in=w384) -> (reference out=w381:refnum<vi>, error out=w383:errorcluster, "FP.State"=w379:T4)
            n172 = Not Equal?(x=w379, y=T4."Closed" ("Front Panel Window:State")) -> (x != y?=w378:bool)
            n173 = case shown="True" w378 {
              tunnel: [w386 w389] -> w385
              tunnel: w383 -> [w386 w388]
              tunnel: w381 -> [_ w387]
              frame False {
              }
              frame True {
                n174 = invoke class="VI" method="FP.Close"(reference=w387, error in=w388) -> (error out=w389:errorcluster)  [unwired: 1 in, 2 out]
              }
            }
          }
          frame "Hidden", "Hide" {
            w390 = T4."Hidden" ("State")
            n175 = property class="VI"(reference=w396, error in=w395) -> (reference out=w393:refnum<vi>, error out=w394:errorcluster, "FP.State"=w392:T4)
            n176 = Not Equal?(x=w392, y=w390) -> (x != y?=w391:bool)
            n177 = case shown="True" w391 {
              tunnel: [w401 w402] -> w397
              tunnel: w394 -> [w400 w402]
              tunnel: w393 -> [w399 _]
              tunnel: w390 -> [w398 _]
              frame True {
                n178 = invoke class="VI" method="FP.Open"(reference=w399, error in=w400, "State"=w398) -> (error out=w401:errorcluster)  [unwired: 2 in, 4 out]
              }
              frame False {
              }
            }
          }
          frame "Minimize", "Minimized" {
            w403 = T4."Minimized" ("State")
            n179 = property class="VI"(reference=w409, error in=w408) -> (reference out=w406:refnum<vi>, error out=w407:errorcluster, "FP.State"=w405:T4)
            n180 = Not Equal?(x=w405, y=w403) -> (x != y?=w404:bool)
            n181 = case shown="True" w404 {
              tunnel: [w414 w415] -> w410
              tunnel: w407 -> [w413 w415]
              tunnel: w406 -> [w412 _]
              tunnel: w403 -> [w411 _]
              frame True {
                n182 = invoke class="VI" method="FP.Open"(reference=w412, error in=w413, "State"=w411) -> (error out=w414:errorcluster)  [unwired: 2 in, 4 out]
              }
              frame False {
              }
            }
          }
          frame "Maximize", "Maximized" {
            w416 = T4."Maximized" ("State")
            n183 = property class="VI"(reference=w422, error in=w421) -> (reference out=w419:refnum<vi>, error out=w420:errorcluster, "FP.State"=w418:T4)
            n184 = Not Equal?(x=w418, y=w416) -> (x != y?=w417:bool)
            n185 = case shown="True" w417 {
              tunnel: [w427 w428] -> w423
              tunnel: w420 -> [w426 w428]
              tunnel: w419 -> [w425 _]
              tunnel: w416 -> [w424 _]
              frame True {
                n186 = invoke class="VI" method="FP.Open"(reference=w425, error in=w426, "State"=w424) -> (error out=w427:errorcluster)  [unwired: 2 in, 4 out]
              }
              frame False {
              }
            }
          }
        }
        n187 = call <vilib>:"Add State(s) to Queue__jki_lib_state_machine.vi"("State(s) in (\"\")"=w363) -> ("States Out"=w362:string)  [unwired: 14 in]
      }
      frame "---------- Macro ----------" {
        # "Do not put any code in this frame.\n(It is a separator no-op. You can make a copy of this frame to create a new Macro frame)"
        n188 = call <vilib>:"Add State(s) to Queue__jki_lib_state_machine.vi"("State(s) in (\"\")"=w433) -> ("States Out"=w432:string)  [unwired: 14 in]
      }
      frame "Macro: Initialize" {
        # "Initialization Macro\n(This is called once, when the VI starts)"
        n189 = call <vilib>:"Add State(s) to Queue__jki_lib_state_machine.vi"("State(s) in Front (\"\")"="Data: Initialize\nInitialize Core Data\nActions: Create and Start Filters\nActions: Load All Binaries\nEvents: Register\nUI: Initialize\nUI: Front Panel State >> Open", "State(s) in (\"\")"=w439) -> ("States Out"=w438:string)  [unwired: 13 in]
      }
      frame "Macro: Exit" {
        # "Exit Macro\n(This is called once, when the VI exits)"
        n190 = Unbundle By Name(w447) -> ("Core.Close Panel on Exit?"=w442:bool)
        n191 = call <vilib>:"Conditional State String__jki_lib_state_machine.vi"("Do State(s)?"=w442, "State"="UI: Front Panel State >> Close") -> ("State Out"=w441:string)  [unwired: 7 in]
        n192 = call <vilib>:"Add State(s) to Queue__jki_lib_state_machine.vi"("State(s) in (\"\")"=w441, "State(s) at Back (\"\")"="UI: Uninitialize\nData: Cleanup\nEvents: Unregister\nExit") -> ("States Out"=w445:string)  [unwired: 13 in]
        n193 = call <vilib>:"Add State(s) to Queue__jki_lib_state_machine.vi"("State(s) in Front (\"\")"=w445, "State(s) in (\"\")"=w449) -> ("States Out"=w448:string)  [unwired: 13 in]
      }
      frame "---------- Actions ----------" {
        # "Template Separator\n(You can make a copy of, or modify, this frame)"
        n194 = call <vilib>:"Add State(s) to Queue__jki_lib_state_machine.vi"("State(s) in (\"\")"=w454) -> ("States Out"=w453:string)  [unwired: 14 in]
      }
      frame "Actions: Create and Start Filters" {
        n195 = control-ref of="team filter"() -> (w478:refnum<vi>)
        n196 = control-ref of="storyArc filter"() -> (w456:refnum<vi>)
        n197 = control-ref of="character filter"() -> (w455:refnum<vi>)
        n198 = control-ref of="concept filter"() -> (w467:refnum<vi>)
        n199 = call "Create.vi"("error in (no error)"=w466, "ref"=w478) -> ("error out"=w477:errorcluster, "selection_dropdown out"=w476:refnum<class "selection_dropdown.lvclass">)  [unwired: 8 in]
        n200 = call "Create.vi"("error in (no error)"=w466, "ref"=w456) -> ("error out"=w472:errorcluster, "selection_dropdown out"=w473:refnum<class "selection_dropdown.lvclass">)  [unwired: 8 in]
        n201 = call "Create.vi"("error in (no error)"=w466, "ref"=w455) -> ("error out"=w471:errorcluster, "selection_dropdown out"=w470:refnum<class "selection_dropdown.lvclass">)  [unwired: 8 in]
        n202 = call "Create.vi"("error in (no error)"=w466, "ref"=w467) -> ("error out"=w468:errorcluster, "selection_dropdown out"=w469:refnum<class "selection_dropdown.lvclass">)  [unwired: 8 in]
        n203 = call "Start.vi"("error in (no error)"=w477, "selection_dropdown in"=w476) -> ("error out"=w457:errorcluster, "selection_dropdown out"=w464:refnum<class "selection_dropdown.lvclass">)  [unwired: 8 in]
        n204 = call "Start.vi"("error in (no error)"=w472, "selection_dropdown in"=w473) -> ("error out"=w458:errorcluster, "selection_dropdown out"=w463:refnum<class "selection_dropdown.lvclass">)  [unwired: 8 in]
        n205 = call "Start.vi"("error in (no error)"=w471, "selection_dropdown in"=w470) -> ("error out"=w459:errorcluster, "selection_dropdown out"=w462:refnum<class "selection_dropdown.lvclass">)  [unwired: 8 in]
        n206 = call "Start.vi"("error in (no error)"=w468, "selection_dropdown in"=w469) -> ("error out"=w460:errorcluster, "selection_dropdown out"=w461:refnum<class "selection_dropdown.lvclass">)  [unwired: 8 in]
        n207 = Bundle By Name(cluster=w465, "filters.team filter"=w464, "filters.story filter"=w463, "filters.char filter"=w462, "filters.concept filter"=w461) -> (w475:T13)
        n208 = Merge Errors(w457, w458, w459, w460) -> (w474:errorcluster)
        n209 = call <vilib>:"Add State(s) to Queue__jki_lib_state_machine.vi"("State(s) in (\"\")"=w481) -> ("States Out"=w480:string)  [unwired: 14 in]
      }
      frame "Actions: Load All Binaries" {
        n210 = call "Load Binaries for Selections.vi"("error in (no error)"=w483, "Cluster in"=w485) -> ("error out"=w482:errorcluster, "Cluster out"=w484:T13)  [unwired: 8 in]
        n211 = call <vilib>:"Add State(s) to Queue__jki_lib_state_machine.vi"("State(s) in (\"\")"=w488) -> ("States Out"=w487:string)  [unwired: 14 in]
      }
      frame "Actions: Zoom All" {
        # "Template Separator\n(You can make a copy of, or modify, this frame)"
        n212 = Unbundle By Name(w495) -> ("picture data.end date"=w490:timestamp, "picture data.start date"=w491:timestamp)
        n213 = property on="Plot Start" class="AbsTime (strict)"(error in=w494, "Val(Sgnl)"=w491) -> (error out=w493:errorcluster)  [unwired: 1 in, 1 out]
        n214 = property on="Plot End" class="AbsTime (strict)"(error in=w493, "Value"=w490) -> (error out=w492:errorcluster)  [unwired: 1 in, 1 out]
        n215 = call <vilib>:"Add State(s) to Queue__jki_lib_state_machine.vi"("State(s) in (\"\")"=w497) -> ("States Out"=w496:string)  [unwired: 14 in]
      }
      frame "Actions: Draw Grid" {
        n216 = property on="2D Picture" class="Pict"(error in=w506) -> (error out=w504:errorcluster, "Draw Area Size"=w505:T19, "Origin"=w498:T20)  [unwired: 1 in, 1 out]
        n217 = local read "Plot Start"() -> (w501:timestamp)
        n218 = local read "Plot End"() -> (w500:timestamp)
        n219 = call "create.grid.vi"("Point"=w498, "Draw Area Size"=w505, "Plot End"=w500, "Plot Start"=w501) -> ("picture"=w503:picture)  [unwired: 7 in]
        n220 = Bundle By Name(cluster=w507, "picture"=w503) -> (w502:T13)
        n221 = call <vilib>:"Add State(s) to Queue__jki_lib_state_machine.vi"("State(s) in (\"\")"=w509) -> ("States Out"=w508:string)  [unwired: 14 in]
      }
      frame "Actions: Display Cursor" {
        n222 = Unbundle By Name(w518) -> ("picture data.names"=w517:string[], "picture data.cells"=w516:T16, "cursor"=w515:T12)
        n223 = for {
          tunnel: w517 -> [w523] mode=indexing
          tunnel: w516 -> [w533] mode=indexing
          tunnel: w515 -> [w528]
          tunnel: [w523] -> w513
          tunnel: [w522] -> w514
          stop <- w522 stop-if-true
          n224 = Unbundle By Name(w528) -> ("Horizontal"=w527:i32, "Vertical"=w526:i32)
          n225 = Unbundle By Name(w533) -> ("right"=w532:i16, "left"=w531:i16, "bottom"=w530:i16, "top"=w529:i16)
          n226 = In Range and Coerce(upper limit=w532, x=w527, lower limit=w531) -> (In Range?=w525:bool)  [unwired: 1 out]
          n227 = In Range and Coerce(upper limit=w530, x=w526, lower limit=w529) -> (In Range?=w524:bool)  [unwired: 1 out]
          n228 = And(x=w525, y=w524) -> (x .and. y?=w522:bool)
        }
        n229 = Select(t=w513, s=w514, f="") -> (s? t:f=→"volume":string)
        n230 = call <vilib>:"Add State(s) to Queue__jki_lib_state_machine.vi"("State(s) in (\"\")"=w521) -> ("States Out"=w520:string)  [unwired: 14 in]
      }
      frame "Actions: Draw Picture" {
        n231 = property on="Legend" class="Clust (strict)"(error in=w536, "Visible"="Show Legend") -> (error out=w535:errorcluster)  [unwired: 1 in, 1 out]
        n232 = call <vilib>:"Add State(s) to Queue__jki_lib_state_machine.vi"("State(s) in (\"\")"=w540) -> ("States Out"=w539:string)  [unwired: 14 in]
      }
      frame "Actions: Build Data" {
        n233 = Unbundle By Name(w556) -> ("manager_daemon"=w557:refnum<class "manager_daemon.lvclass">, "filters.team filter"=w548:refnum<class "selection_dropdown.lvclass">, "filters.char filter"=w544:refnum<class "selection_dropdown.lvclass">, "filters.story filter"=w545:refnum<class "selection_dropdown.lvclass">, "filters.concept filter"=w546:refnum<class "selection_dropdown.lvclass">)
        n234 = call "Filter List.get.vi"("selection_dropdown in"=w548) -> ("filter list"=w547:string[])  [unwired: 9 in, 1 out]
        n235 = call "Filter List.get.vi"("selection_dropdown in"=w544) -> ("filter list"=w541:string[])  [unwired: 9 in, 1 out]
        n236 = call "Filter List.get.vi"("selection_dropdown in"=w545) -> ("filter list"=w542:string[])  [unwired: 9 in, 1 out]
        n237 = call "Filter List.get.vi"("selection_dropdown in"=w546) -> ("filter list"=w543:string[])  [unwired: 9 in, 1 out]
        n238 = local read "Plot Start"() -> (w561:timestamp)
        n239 = local read "Plot End"() -> (w562:timestamp)
        n240 = Bundle(cluster=T6 {"Volume Type"={"Ongoing"=TRUE, "Limited Series"=TRUE, "Annuals"=TRUE, "One Shots"=TRUE, "Reference/Reprints"=TRUE, "Star Comics"=TRUE, "Epic Comics"=TRUE}, "team"=[], "characters"=[], "storyArcs"=[], "Plot End"=timestamp(0 s since 1904-01-01), "Plot Start"=timestamp(0 s since 1904-01-01), "title"=[], "colors"={"ongoing"=0, "Limited Series"=0, "Annuals"=0, "One Shots"=0, "Reprints"=0, "Star"=0, "Epic"=0}, "concept"=[], "show all"=FALSE, "Search by Title"=enum."AND"} ("selection filter"), "Volume Type"="Volume Type", "team"=w547, "characters"=w541, "storyArcs"=w542, "Plot End"=w562, "Plot Start"=w561, "title"="title", "colors"="Legend", "concept"=w543, "show all"="Show All", "Search by Title"="Apply Filters") -> (w551:T6)
        n241 = call "filter data.vi"("graph only (f)"=TRUE, "error in (no error)"=w554, "selection filter"=w551, "manager_daemon in"=w557) -> ("error out"=w555:errorcluster)  [unwired: 6 in, 1 out]
        n242 = call <vilib>:"Add State(s) to Queue__jki_lib_state_machine.vi"("State(s) in (\"\")"=w565) -> ("States Out"=w564:string)  [unwired: 14 in]
      }
      frame "Actions: Calculate Rows" {
        w567 = 16  # Row Height
        w568 = 32  # Row Height
        n243 = Unbundle By Name(w573) -> ("volume objects"=w576:cluster{"Array":T8[]}[])
        n244 = local read "Show Issues"() -> (w569:bool)
        n245 = Array Size(array=w576) -> (size(s)=w575:i32)
        n246 = Select(t=w568, s=w569, f=w567) -> (s? t:f=w566:i32)
        n247 = for {
          N: w575 -> [_]
          tunnel: T7 {"left"=0, "top"=0, "right"=0, "bottom"=0} ("rect") -> [w587]
          tunnel: [w586] -> w571 mode=indexing
          tunnel: w566 -> [w583]
          i -> [w585]
          n248 = Multiply(x=w583, y=w585) -> (x*y=w584:i32)
          n249 = Add(x=w584, y=w583) -> (x+y=w582:i32)
          n250 = Subtract(x=w582, y=2) -> (x-y=w580:i32)
          n251 = Bundle By Name(cluster=w587, "top"=w584, "bottom"=w580) -> (w586:T7)
        }
        n252 = Bundle By Name(cluster=w573, "rows"=w571) -> (w572:T13)
        n253 = call <vilib>:"Add State(s) to Queue__jki_lib_state_machine.vi"("State(s) in (\"\")"=w579) -> ("States Out"=w578:string)  [unwired: 14 in]
      }
      frame "Actions: Calculate Cells" {
        n254 = Unbundle By Name(w594) -> ("picture"=w595:picture, "volume objects"=w600:cluster{"Array":T8[]}[], "rows"=w599:T16)
        n255 = property on="2D Picture" class="Pict"() -> ("Draw Area Size"=w601:T19)  [unwired: 2 in, 2 out]
        n256 = Unbundle By Name(w601) -> ("Width"=w598:u32)
        n257 = local read "Plot Start"() -> (w597:timestamp)
        n258 = local read "Plot End"() -> (w596:timestamp)
        n259 = call "plot.volumes.vi"("plot end"=w596, "Show Issues"="Show Issues", "plot start"=w597, "picture in"=w595, "Width"=w598, "rows"=w599, "volume objects"=w600) -> ("names"=w590:string[], "cells"=w591:T16, "picture"=w592:picture)  [unwired: 2 in]
        "2D Picture" <- w592
        n260 = Bundle By Name(cluster=w594, "picture"=w592, "picture data.cells"=w591, "picture data.names"=w590) -> (w593:T13)
      }
    }
  }
